vi "Lab Panel V5.0.vi"() -> ()   [LabVIEW 2013] (continued)
                      tunnel: w2669 -> [_ w2673]
                      frame False {
                      }
                      frame True {
                        n1581 = stacked-sequence {
                          tunnel: w2674 -> [w2677 _ _]
                          tunnel: w2673 -> [_ w2679 _]
                          frame #0 {
                            w2675 = FALSE
                            n1582 = local write "mail control"("END") -> ()
                            n1583 = Bundle(cluster=w2677) -> (w2678:T4)  [unwired: 3 in]
                            n1584 = local write "O/I  LAB05-1"(w2675) -> ()
                            n1585 = local write "RUN LAB05-1"(w2675) -> ()
                            n1586 = local write "run lab05-1"(w2675) -> ()
                            n1587 = local write "DISP LAB05-1"(w2678) -> ()
                          }
                          frame #1 {
                            n1588 = TDMS Close(11:w2679) -> (0:w2680:errorcluster)  [unwired: 1 in, 1 out]
                            n1589 = local write "data file error"(w2680) -> ()
                          }
                          frame #2 {
                            n1590 = stacked-sequence {
                              tunnel: "LAB05-1" -> [w2683 w2685]
                              frame #0 {
                                n1591 = call "sub vi - defrag tdms v1.vi"("panel id"=w2683) -> ("error out"=w2682:errorcluster)  [unwired: 10 in]
                                n1592 = local write "data file error"(w2682) -> ()
                              }
                              frame #1 {
                                n1593 = call "Save data file to network drive v2.vi"("panel id"=w2685) -> ("network file save error"=w2684:errorcluster)  [unwired: 9 in, 1 out]
                                n1594 = local write "data file error"(w2684) -> ()
                              }
                            }
                          }
                        }
                      }
                    }
                  }
                }
              }
              frame #9 {
                # "LAB05-2"
                n1595 = local read "run lab05-2"() -> (w2686:bool)
                n1596 = case shown="True" w2686 {
                  frame False {
                  }
                  frame True {
                    n1597 = local read "DISP LAB05-2"() -> (w2693:T4)
                    n1598 = Unbundle(w2693) -> ("CYCLE"=w2689:dbl, "STATUS"=w2694:string)  [unwired: 1 out]
                    n1599 = Not Equal?(x=w2694, y="RUN") -> (x != y?=w2688:bool)
                    n1600 = local read "TDMS LAB05-2"() -> (w2692:refnum<k34>)
                    n1601 = Greater?(x=w2689, y=2.0) -> (0:w2690:bool)
                    n1602 = And(x=w2690, y=w2688) -> (x .and. y?=w2687:bool)
                    n1603 = case shown="True" w2687 {
                      tunnel: w2693 -> [_ w2697]
                      tunnel: w2692 -> [_ w2696]
                      frame False {
                      }
                      frame True {
                        n1604 = stacked-sequence {
                          tunnel: w2697 -> [w2700 _ _]
                          tunnel: w2696 -> [_ w2702 _]
                          frame #0 {
                            w2698 = FALSE
                            n1605 = local write "mail control"("END") -> ()
                            n1606 = Bundle(cluster=w2700) -> (w2701:T4)  [unwired: 3 in]
                            n1607 = local write "RUN LAB05-2"(w2698) -> ()
                            n1608 = local write "O/I  LAB05-2"(w2698) -> ()
                            n1609 = local write "run lab05-2"(w2698) -> ()
                            n1610 = local write "DISP LAB05-2"(w2701) -> ()
                          }
                          frame #1 {
                            n1611 = TDMS Close(11:w2702) -> (0:w2703:errorcluster)  [unwired: 1 in, 1 out]
                            n1612 = local write "data file error"(w2703) -> ()
                          }
                          frame #2 {
                            n1613 = stacked-sequence {
                              tunnel: "LAB05-2" -> [w2706 w2708]
                              frame #0 {
                                n1614 = call "sub vi - defrag tdms v1.vi"("panel id"=w2706) -> ("error out"=w2705:errorcluster)  [unwired: 10 in]
                                n1615 = local write "data file error"(w2705) -> ()
                              }
                              frame #1 {
                                n1616 = call "Save data file to network drive v2.vi"("panel id"=w2708) -> ("network file save error"=w2707:errorcluster)  [unwired: 9 in, 1 out]
                                n1617 = local write "data file error"(w2707) -> ()
                              }
                            }
                          }
                        }
                      }
                    }
                  }
                }
              }
            }
            n1618 = local read "Network Directory"() -> (w2462:path)
            n1619 = global write "Global 1.vi" "Network Drive"(w2462) -> ()
          }
          frame #7 {
            # "disable functions"
            n1620 = stacked-sequence {
              tunnel: w2718 -> [w2732 _ w2789]
              tunnel: w2717 -> [w2727 _ w2788]
              tunnel: w2716 -> [w2726 _ w2787]
              tunnel: w2715 -> [w2724 _ w2786]
              tunnel: w2714 -> [w2725 _ w2785]
              tunnel: w2713 -> [_ w2749 w2784]
              tunnel: w2712 -> [_ w2750 w2783]
              tunnel: w2711 -> [_ w2751 w2782]
              tunnel: w2710 -> [_ w2752 w2781]
              tunnel: w2709 -> [_ w2753 w2780]
              frame #0 {
                n1621 = Select(t=2, s=w2724, f=0) -> (s? t:f=w2720:i32)
                n1622 = Select(t=2, s=w2726, f=0) -> (s? t:f=w2721:i32)
                n1623 = Select(t=2, s=w2725, f=0) -> (s? t:f=w2719:i32)
                n1624 = Select(t=2, s=w2732, f=0) -> (s? t:f=w2723:i32)
                n1625 = Select(t=2, s=w2727, f=0) -> (s? t:f=w2722:i32)
                n1626 = property on="SELECT LAB02-2" class="RadioBtnsControl (strict)"("DisabledEnum"=w2720) -> ()  [unwired: 2 in, 2 out]
                n1627 = property on="SELECT LAB02-1" class="RadioBtnsControl (strict)"("DisabledEnum"=w2721) -> ()  [unwired: 2 in, 2 out]
                n1628 = property on="SELECT LAB03-1" class="RadioBtnsControl (strict)"("DisabledEnum"=w2719) -> ()  [unwired: 2 in, 2 out]
                n1629 = property on="SELECT LAB01-1" class="RadioBtnsControl (strict)"("DisabledEnum"=w2723) -> ()  [unwired: 2 in, 2 out]
                n1630 = property on="SELECT LAB01-2" class="RadioBtnsControl (strict)"("DisabledEnum"=w2722) -> ()  [unwired: 2 in, 2 out]
                n1631 = Not(x=w2732) -> (.not. x?=w2733:bool)
                n1632 = property on="RESULT LAB01-1" class="Bool (strict)"("Visible"=w2733) -> ()  [unwired: 2 in, 2 out]
                n1633 = Not(x=w2727) -> (.not. x?=w2731:bool)
                n1634 = Not(x=w2726) -> (.not. x?=w2730:bool)
                n1635 = Not(x=w2724) -> (.not. x?=w2729:bool)
                n1636 = property on="RESULT LAB01-2" class="Bool (strict)"("Visible"=w2731) -> ()  [unwired: 2 in, 2 out]
                n1637 = Not(x=w2725) -> (.not. x?=w2728:bool)
                n1638 = property on="RESULT LAB02-1" class="Bool (strict)"("Visible"=w2730) -> ()  [unwired: 2 in, 2 out]
                n1639 = property on="RESULT LAB02-2" class="Bool (strict)"("Visible"=w2729) -> ()  [unwired: 2 in, 2 out]
                n1640 = property on="RESULT LAB03-1" class="Bool (strict)"("Visible"=w2728) -> ()  [unwired: 2 in, 2 out]
                n1641 = property on="SET LAB01-1" class="Clust (strict)"("DisabledEnum"=w2723) -> ()  [unwired: 2 in, 2 out]
                n1642 = property on="SET LAB01-2" class="Clust (strict)"("DisabledEnum"=w2722) -> ()  [unwired: 2 in, 2 out]
                n1643 = property on="SET LAB02-1" class="Clust (strict)"("DisabledEnum"=w2721) -> ()  [unwired: 2 in, 2 out]
                n1644 = property on="SET LAB02-2" class="Clust (strict)"("DisabledEnum"=w2720) -> ()  [unwired: 2 in, 2 out]
                n1645 = property on="SET LAB03-1" class="Clust (strict)"("DisabledEnum"=w2719) -> ()  [unwired: 2 in, 2 out]
                n1646 = property on="O/I  LAB01-1" class="Bool (strict)"("DisabledEnum"=w2723) -> ()  [unwired: 2 in, 2 out]
                n1647 = property on="O/I  LAB01-2" class="Bool (strict)"("DisabledEnum"=w2722) -> ()  [unwired: 2 in, 2 out]
                n1648 = property on="O/I  LAB02-1" class="Bool (strict)"("DisabledEnum"=w2721) -> ()  [unwired: 2 in, 2 out]
                n1649 = property on="O/I  LAB02-2" class="Bool (strict)"("DisabledEnum"=w2720) -> ()  [unwired: 2 in, 2 out]
                n1650 = property on="O/I  LAB03-1" class="Bool (strict)"("DisabledEnum"=w2719) -> ()  [unwired: 2 in, 2 out]
              }
              frame #1 {
                n1651 = Select(t=2, s=w2753, f=0) -> (s? t:f=w2744:i32)
                n1652 = Select(t=2, s=w2752, f=0) -> (s? t:f=w2745:i32)
                n1653 = Select(t=2, s=w2749, f=0) -> (s? t:f=w2748:i32)
                n1654 = Select(t=2, s=w2750, f=0) -> (s? t:f=w2747:i32)
                n1655 = Select(t=2, s=w2751, f=0) -> (s? t:f=w2746:i32)
                n1656 = property on="SELECT LAB05-2" class="RadioBtnsControl (strict)"("DisabledEnum"=w2744) -> ()  [unwired: 2 in, 2 out]
                n1657 = property on="SELECT LAB05-1" class="RadioBtnsControl (strict)"("DisabledEnum"=w2745) -> ()  [unwired: 2 in, 2 out]
                n1658 = property on="SELECT LAB03-2" class="RadioBtnsControl (strict)"("DisabledEnum"=w2748) -> ()  [unwired: 2 in, 2 out]
                n1659 = property on="SELECT LAB04-1" class="RadioBtnsControl (strict)"("DisabledEnum"=w2747) -> ()  [unwired: 2 in, 2 out]
                n1660 = property on="SELECT LAB04-2" class="RadioBtnsControl (strict)"("DisabledEnum"=w2746) -> ()  [unwired: 2 in, 2 out]
                n1661 = property on="SET LAB05-2" class="Clust (strict)"("DisabledEnum"=w2744) -> ()  [unwired: 2 in, 2 out]
                n1662 = property on="SET LAB05-1" class="Clust (strict)"("DisabledEnum"=w2745) -> ()  [unwired: 2 in, 2 out]
                n1663 = property on="SET LAB03-2" class="Clust (strict)"("DisabledEnum"=w2748) -> ()  [unwired: 2 in, 2 out]
                n1664 = property on="SET LAB04-1" class="Clust (strict)"("DisabledEnum"=w2747) -> ()  [unwired: 2 in, 2 out]
                n1665 = property on="SET LAB04-2" class="Clust (strict)"("DisabledEnum"=w2746) -> ()  [unwired: 2 in, 2 out]
                n1666 = property on="O/I  LAB05-2" class="Bool (strict)"("DisabledEnum"=w2744) -> ()  [unwired: 2 in, 2 out]
                n1667 = property on="O/I  LAB05-1" class="Bool (strict)"("DisabledEnum"=w2745) -> ()  [unwired: 2 in, 2 out]
                n1668 = property on="O/I  LAB04-1" class="Bool (strict)"("DisabledEnum"=w2747) -> ()  [unwired: 2 in, 2 out]
                n1669 = property on="O/I  LAB04-2" class="Bool (strict)"("DisabledEnum"=w2746) -> ()  [unwired: 2 in, 2 out]
                n1670 = property on="O/I  LAB03-2" class="Bool (strict)"("DisabledEnum"=w2748) -> ()  [unwired: 2 in, 2 out]
                n1671 = Not(x=w2753) -> (.not. x?=w2754:bool)
                n1672 = Not(x=w2752) -> (.not. x?=w2755:bool)
                n1673 = Not(x=w2751) -> (.not. x?=w2756:bool)
                n1674 = property on="RESULT LAB05-2" class="Bool (strict)"("Visible"=w2754) -> ()  [unwired: 2 in, 2 out]
                n1675 = property on="RESULT LAB05-1" class="Bool (strict)"("Visible"=w2755) -> ()  [unwired: 2 in, 2 out]
                n1676 = Not(x=w2750) -> (.not. x?=w2757:bool)
                n1677 = property on="RESULT LAB04-2" class="Bool (strict)"("Visible"=w2756) -> ()  [unwired: 2 in, 2 out]
                n1678 = Not(x=w2749) -> (.not. x?=w2758:bool)
                n1679 = property on="RESULT LAB04-1" class="Bool (strict)"("Visible"=w2757) -> ()  [unwired: 2 in, 2 out]
                n1680 = property on="RESULT LAB03-2" class="Bool (strict)"("Visible"=w2758) -> ()  [unwired: 2 in, 2 out]
              }
              frame #2 {
                # "disable calibrate if any test running"
                n1681 = Or(x=w2781, y=w2780) -> (x .or. y?=w2774:bool)
                n1682 = Or(x=w2783, y=w2782) -> (x .or. y?=w2776:bool)
                n1683 = Or(x=w2787, y=w2786) -> (x .or. y?=w2778:bool)
                n1684 = Or(x=w2785, y=w2784) -> (x .or. y?=w2777:bool)
                n1685 = Or(x=w2789, y=w2788) -> (x .or. y?=w2779:bool)
                n1686 = Or(x=w2777, y=w2776) -> (x .or. y?=w2775:bool)
                n1687 = Or(x=w2779, y=w2778) -> (x .or. y?=w2773:bool)
                n1688 = Or(x=w2775, y=w2774) -> (x .or. y?=w2772:bool)
                n1689 = Or(x=w2773, y=w2772) -> (x .or. y?=w2771:bool)
                n1690 = case shown="False" w2771 {
                  tunnel: [0 2] -> w2770
                  frame False {
                  }
                  frame True {
                  }
                }
                n1691 = property on="JIG TEST" class="Clust (strict)"("DisabledEnum"=w2770) -> ()  [unwired: 2 in, 2 out]
                n1692 = property on="Network Directory" class="Path"("DisabledEnum"=w2770) -> ()  [unwired: 2 in, 2 out]
                n1693 = property on="MAIL SETTINGS" class="Clust (strict)"("DisabledEnum"=w2770) -> ()  [unwired: 2 in, 2 out]
                n1694 = property on="SET (cal)" class="Bool (strict)"("DisabledEnum"=w2770) -> ()  [unwired: 2 in, 2 out]
                n1695 = property on="ADMIN" class="Bool (strict)"("DisabledEnum"=0) -> ()  [unwired: 2 in, 2 out]
              }
            }
          }
          frame #8 {
            # "drive jigs"
            n1696 = stacked-sequence {
              frame #0 {
                # "jig on"
                n1697 = local read "jig cycle"() -> (w2797:dbl)
                n1698 = property on="JIG TEST" class="Clust (strict)"() -> ("DisabledEnum"=w2794:T14)  [unwired: 2 in, 2 out]
                n1699 = Equal?(x=w2794, y=2) -> (x = y?=w2793:bool)
                n1700 = Equal?(x=w2797, y=0) -> (x = y?=w2795:bool)
                n1701 = And(x=w2795, y=w2793) -> (x .and. y?=w2792:bool)
                n1702 = case shown="True" w2792 {
                  frame False {
                  }
                  frame True {
                    n1703 = local read "run lab01-1"() -> (w2808:bool)
                    n1704 = local read "run lab01-2"() -> (w2807:bool)
                    n1705 = local read "run lab02-1"() -> (w2806:bool)
                    n1706 = local read "run lab02-2"() -> (w2805:bool)
                    n1707 = local read "run lab03-1"() -> (w2804:bool)
                    n1708 = local read "run lab03-2"() -> (w2803:bool)
                    n1709 = local read "run lab04-1"() -> (w2802:bool)
                    n1710 = local read "run lab04-2"() -> (w2801:bool)
                    n1711 = local read "run lab05-1"() -> (w2800:bool)
                    n1712 = local read "run lab05-2"() -> (w2799:bool)
                    n1713 = local write "JIG LAB03-2"(w2803) -> ()
                    n1714 = local write "JIG LAB01-1"(w2808) -> ()
                    n1715 = local write "JIG LAB01-2"(w2807) -> ()
                    n1716 = local write "JIG LAB02-1"(w2806) -> ()
                    n1717 = local write "JIG LAB02-2"(w2805) -> ()
                    n1718 = local write "JIG LAB03-1"(w2804) -> ()
                    n1719 = local write "JIG LAB04-1"(w2802) -> ()
                    n1720 = local write "JIG LAB04-2"(w2801) -> ()
                    n1721 = local write "JIG LAB05-1"(w2800) -> ()
                    n1722 = local write "JIG LAB05-2"(w2799) -> ()
                  }
                }
              }
              frame #1 {
                # "jig off"
                n1723 = local read "jig cycle"() -> (w2815:dbl)
                n1724 = local read "on loops"() -> (w2814:dbl)
                n1725 = property on="JIG TEST" class="Clust (strict)"() -> ("DisabledEnum"=w2813:T14)  [unwired: 2 in, 2 out]
                n1726 = Equal?(x=w2813, y=2) -> (x = y?=w2811:bool)
                n1727 = Equal?(x=w2815, y=w2814) -> (x = y?=w2810:bool)
                n1728 = And(x=w2810, y=w2811) -> (x .and. y?=w2809:bool)
                n1729 = case shown="True" w2809 {
                  frame False {
                  }
                  frame True {
                    w2866 = FALSE
                    w2867 = TRUE
                    w2865 = 2
                    n1730 = local read "SELECT LAB05-2"() -> (w2856:T3)
                    n1731 = local read "SELECT LAB04-2"() -> (w2858:T3)
                    n1732 = local read "SELECT LAB04-1"() -> (w2859:T3)
                    n1733 = local read "SELECT LAB05-1"() -> (w2857:T3)
                    n1734 = local read "SELECT LAB03-2"() -> (w2860:T3)
                    n1735 = local read "SELECT LAB02-1"() -> (w2863:T3)
                    n1736 = local read "SELECT LAB03-1"() -> (w2861:T3)
                    n1737 = local read "SELECT LAB02-2"() -> (w2862:T3)
                    n1738 = local read "SELECT LAB01-2"() -> (w2864:T3)
                    n1739 = local read "run lab05-1"() -> (w2826:bool)
                    n1740 = local read "run lab05-2"() -> (w2825:bool)
                    n1741 = local read "SELECT LAB01-1"() -> (w2868:T3)
                    n1742 = local read "run lab04-2"() -> (w2827:bool)
                    n1743 = local read "run lab04-1"() -> (w2828:bool)
                    n1744 = local read "run lab01-1"() -> (w2844:bool)
                    n1745 = local read "run lab01-2"() -> (w2833:bool)
                    n1746 = local read "run lab03-2"() -> (w2829:bool)
                    n1747 = local read "run lab03-1"() -> (w2830:bool)
                    n1748 = local read "run lab02-1"() -> (w2832:bool)
                    n1749 = local read "run lab02-2"() -> (w2831:bool)
                    n1750 = Equal?(x=w2865, y=w2861) -> (x = y?=w2839:bool)
                    n1751 = Equal?(x=w2865, y=w2860) -> (x = y?=w2838:bool)
                    n1752 = Equal?(x=w2865, y=w2859) -> (x = y?=w2837:bool)
                    n1753 = Equal?(x=w2865, y=w2858) -> (x = y?=w2836:bool)
                    n1754 = Equal?(x=w2865, y=w2857) -> (x = y?=w2835:bool)
                    n1755 = Equal?(x=w2865, y=w2856) -> (x = y?=w2834:bool)
                    n1756 = Equal?(x=w2865, y=w2868) -> (x = y?=w2845:bool)
                    n1757 = Equal?(x=w2865, y=w2863) -> (x = y?=w2841:bool)
                    n1758 = Equal?(x=w2865, y=w2862) -> (x = y?=w2840:bool)
                    n1759 = Equal?(x=w2865, y=w2864) -> (x = y?=w2842:bool)
                    n1760 = And(x=w2836, y=w2827) -> (x .and. y?=w2818:bool)
                    n1761 = And(x=w2839, y=w2830) -> (x .and. y?=w2821:bool)
                    n1762 = And(x=w2837, y=w2828) -> (x .and. y?=w2819:bool)
                    n1763 = And(x=w2834, y=w2825) -> (x .and. y?=w2816:bool)
                    n1764 = And(x=w2840, y=w2831) -> (x .and. y?=w2822:bool)
                    n1765 = And(x=w2838, y=w2829) -> (x .and. y?=w2820:bool)
                    n1766 = And(x=w2835, y=w2826) -> (x .and. y?=w2817:bool)
                    n1767 = And(x=w2842, y=w2833) -> (x .and. y?=w2824:bool)
                    n1768 = And(x=w2845, y=w2844) -> (x .and. y?=w2843:bool)
                    n1769 = And(x=w2841, y=w2832) -> (x .and. y?=w2823:bool)
                    n1770 = Select(t=w2867, s=w2843, f=w2866) -> (s? t:f=w2846:bool)
                    n1771 = Select(t=w2867, s=w2824, f=w2866) -> (s? t:f=w2847:bool)
                    n1772 = Select(t=w2867, s=w2823, f=w2866) -> (s? t:f=w2848:bool)
                    n1773 = Select(t=w2867, s=w2822, f=w2866) -> (s? t:f=w2849:bool)
                    n1774 = Select(t=w2867, s=w2821, f=w2866) -> (s? t:f=w2850:bool)
                    n1775 = Select(t=w2867, s=w2820, f=w2866) -> (s? t:f=w2851:bool)
                    n1776 = Select(t=w2867, s=w2819, f=w2866) -> (s? t:f=w2852:bool)
                    n1777 = Select(t=w2867, s=w2818, f=w2866) -> (s? t:f=w2853:bool)
                    n1778 = Select(t=w2867, s=w2817, f=w2866) -> (s? t:f=w2854:bool)
                    n1779 = Select(t=w2867, s=w2816, f=w2866) -> (s? t:f=w2855:bool)
                    n1780 = local write "JIG LAB03-2"(w2851) -> ()
                    n1781 = local write "JIG LAB02-1"(w2848) -> ()
                    n1782 = local write "JIG LAB02-2"(w2849) -> ()
                    n1783 = local write "JIG LAB01-2"(w2847) -> ()
                    n1784 = local write "JIG LAB03-1"(w2850) -> ()
                    n1785 = local write "JIG LAB01-1"(w2846) -> ()
                    n1786 = local write "JIG LAB05-2"(w2855) -> ()
                    n1787 = local write "JIG LAB04-1"(w2852) -> ()
                    n1788 = local write "JIG LAB05-1"(w2854) -> ()
                    n1789 = local write "JIG LAB04-2"(w2853) -> ()
                  }
                }
              }
            }
          }
          frame #9 {
            # "enable  jig test output if no test busy"
            n1790 = property on="JIG TEST" class="Clust (strict)"() -> ("DisabledEnum"=w2871:T14)  [unwired: 2 in, 2 out]
            n1791 = Equal?(x=w2871, y=0) -> (x = y?=w2869:bool)
            n1792 = case shown="True" w2869 {
              frame False {
              }
              frame True {
                n1793 = local read "JIG TEST"() -> (w2882:T9)
                n1794 = Unbundle(w2882) -> ("LAB01-1"=w2881:bool, "LAB01-2"=w2880:bool, "LAB02-1"=w2879:bool, "LAB02-2"=w2878:bool, "LAB03-1"=w2877:bool, "LAB03-2"=w2876:bool, "LAB04-1"=w2875:bool, "LAB04-2"=w2874:bool, "LAB05-1"=w2873:bool, "LAB05-2"=w2872:bool)
                n1795 = local write "JIG LAB05-1"(w2873) -> ()
                n1796 = local write "JIG LAB05-2"(w2872) -> ()
                n1797 = local write "JIG LAB04-1"(w2875) -> ()
                n1798 = local write "JIG LAB04-2"(w2874) -> ()
                n1799 = local write "JIG LAB03-2"(w2876) -> ()
                n1800 = local write "JIG LAB01-1"(w2881) -> ()
                n1801 = local write "JIG LAB02-1"(w2879) -> ()
                n1802 = local write "JIG LAB03-1"(w2877) -> ()
                n1803 = local write "JIG LAB01-2"(w2880) -> ()
                n1804 = local write "JIG LAB02-2"(w2878) -> ()
              }
            }
          }
          frame #10 {
            # "drive digital output"
            n1805 = local read "O/I  LAB05-2"() -> (w2889:bool)
            n1806 = local read "O/I  LAB05-1"() -> (w2891:bool)
            n1807 = local read "JIG LAB05-2"() -> (w2888:bool)
            n1808 = local read "O/I  LAB04-2"() -> (w2893:bool)
            n1809 = local read "JIG LAB05-1"() -> (w2890:bool)
            n1810 = local read "JIG LAB04-2"() -> (w2892:bool)
            n1811 = local read "O/I  LAB03-1"() -> (w2898:bool)
            n1812 = local read "O/I  LAB04-1"() -> (w2894:bool)
            n1813 = local read "O/I  LAB02-1"() -> (w2902:bool)
            n1814 = local read "O/I  LAB02-2"() -> (w2900:bool)
            n1815 = local read "O/I  LAB03-2"() -> (w2896:bool)
            n1816 = local read "JIG LAB04-1"() -> (w2887:bool)
            n1817 = local read "JIG LAB03-2"() -> (w2895:bool)
            n1818 = local read "O/I  LAB01-2"() -> (w2904:bool)
            n1819 = local read "JIG LAB02-1"() -> (w2901:bool)
            n1820 = local read "JIG LAB02-2"() -> (w2899:bool)
            n1821 = local read "JIG LAB03-1"() -> (w2897:bool)
            n1822 = local read "O/I  LAB01-1"() -> (w2906:bool)
            n1823 = local read "JIG LAB01-2"() -> (w2903:bool)
            n1824 = local read "JIG LAB01-1"() -> (w2905:bool)
            n1825 = Build Array(w2893, w2892, w2891, w2890, w2889, w2888) -> (w2884:bool[])
            n1826 = Build Array(w2899, w2898, w2897, w2896, w2895, w2894, w2887) -> (w2885:bool[])
            n1827 = Build Array(w2906, w2905, w2904, w2903, w2902, w2901, w2900) -> (w2886:bool[])
            n1828 = local read "simulate"() -> (w2883:bool)
            n1829 = case shown="False" w2883 {
              tunnel: w2886 -> [w2909 _]
              tunnel: w2885 -> [w2908 _]
              tunnel: w2884 -> [w2907 _]
              frame False {
                n1830 = call "sub vi - Drive Relays All v6.vi"("Array #2"=w2907, "Array #1"=w2908, "Array #0"=w2909) -> ()  [unwired: 8 in, 1 out]
              }
              frame True {
              }
            }
          }
          frame #11 {
            # "get analog values"
            n1831 = local read "on loops"() -> (w2916:dbl)
            n1832 = local read "jig cycle"() -> (w2913:dbl)
            n1833 = Add(x=w2916, y=1) -> (x+y=w2914:dbl)
            n1834 = Equal?(x=w2913, y=1) -> (x = y?=w2911:bool)
            n1835 = Equal?(x=w2913, y=w2914) -> (x = y?=w2912:bool)
            n1836 = Or(x=w2911, y=w2912) -> (x .or. y?=w2910:bool)
            n1837 = case shown="True" w2910 {
              frame False {
              }
              frame True {
                n1838 = local read "simulate"() -> (w2920:bool)
                n1839 = case shown="False" w2920 {
                  tunnel: [w2936 errorcluster[] [] ("array ERROR")] -> w2928
                  tunnel: [w2935 0.3 ("Analog loop time")] -> w2927
                  tunnel: [w2934 dynamicdata[] [] ("array GRAPH")] -> w2926
                  tunnel: [w2933 w2938] -> w2925
                  tunnel: [w2932 w2938] -> w2924
                  tunnel: [w2931 w2938] -> w2923
                  tunnel: [w2930 w2938] -> w2922
                  tunnel: [w2929 w2938] -> w2921
                  frame False {
                    n1840 = call "sub vi - Read Analog All v8.vi"() -> ("Analog loop time"=w2935:dbl, "array GRAPH"=w2934:dynamicdata[], "LAB01"=w2933:T23, "LAB02"=w2932:T24, "LAB03"=w2931:T25, "LAB04"=w2930:T26, "array ERROR"=w2936:errorcluster[], "LAB05"=w2929:T27)  [unwired: 7 in, 1 out]
                  }
                  frame True {
                    w2938 = T27 {"LAB05-1 (A)"=10.0, "LAB05-1 (V)"=220.0, "LAB05-1 (PF)"=0.5, "LAB05-2 (A)"=15.0, "LAB05-2 (V)"=225.0, "LAB05-2 (PF)"=0.6} ("LAB05")
                  }
                }
                n1841 = local read "simulate"() -> (w2919:bool)
                n1842 = stacked-sequence {
                  tunnel: w2928 -> [w2945 _ _ _ _ _]
                  tunnel: w2927 -> [w2944 _ _ _ _ _]
                  tunnel: w2926 -> [w2943 _ _ _ _ _]
                  tunnel: w2925 -> [_ w2992 _ _ _ _]
                  tunnel: w2924 -> [_ _ w2999 _ _ _]
                  tunnel: w2923 -> [_ _ _ w3028 _ _]
                  tunnel: w2922 -> [_ _ _ _ w3055 _]
                  tunnel: w2921 -> [_ _ _ _ _ w3084]
                  tunnel: w2919 -> [_ w2970 w2998 w3026 w3054 w3082]
                  tunnel: T12 {"1  (A) cal"=1.0, "1 (V) cal"=1.0, "1 (PF) cal"=1.0, "1 (TL) cal"=1.0, "1 (TN) cal"=1.0, "2 (A) cal"=1.0, "2 (V) cal"=1.0, "2 (PF) cal"=1.0, "2 (TL) cal"=1.0, "2 (TN) cal"=1.0} ("CAL LAB01") -> [_ w2969 w2997 w3025 w3053 w3081]
                  frame #0 {
                    n1843 = local write "AI"(TRUE) -> ()
                    n1844 = global write "Global 1.vi" "RATE(Hz)"("RATE (Hz)") -> ()
                    n1845 = global write "Global 1.vi" "SAMPLES"("SAMPLES") -> ()
                    n1846 = Index Array(array=w2943, index=6) -> (element=→"LAB04-1 (GRAPH)":dynamicdata)
                    n1847 = Index Array(array=w2943, index=7) -> (element=→"LAB04-2 (GRAPH)":dynamicdata)
                    n1848 = Index Array(array=w2943, index=9) -> (element=→"LAB05-2 (GRAPH)":dynamicdata)
                    n1849 = Index Array(array=w2943, index=8) -> (element=→"LAB05-1 (GRAPH)":dynamicdata)
                    n1850 = Index Array(array=w2943, index=5) -> (element=→"LAB03-2 (GRAPH)":dynamicdata)
                    n1851 = Index Array(array=w2943, index=0) -> (element=→"LAB01-1 (GRAPH)":dynamicdata)
                    n1852 = Index Array(array=w2943, index=1) -> (element=→"LAB01-2 (GRAPH)":dynamicdata)
                    n1853 = Index Array(array=w2943, index=2) -> (element=→"LAB02-1 (GRAPH)":dynamicdata)
                    n1854 = Index Array(array=w2943, index=3) -> (element=→"LAB02-2 (GRAPH)":dynamicdata)
                    n1855 = Index Array(array=w2943, index=4) -> (element=→"LAB03-1 (GRAPH)":dynamicdata)
                    "AI loop time" <- w2944
                    "Analog Error Array" <- w2945
                  }
                  frame #1 {
                    n1856 = Unbundle By Name(w2992) -> ("LAB05-1 (A)"=w2990:dbl, "LAB05-1 (V)"=w2989:dbl, "LAB05-1 (PF)"=w2988:dbl, "LAB05-2 (A)"=w2987:dbl, "LAB05-2 (V)"=w2986:dbl, "LAB05-2 (PF)"=w2985:dbl)
                    n1857 = case shown="False" w2970 {
                      tunnel: [w2993 w2994] -> w2991
                      tunnel: w2969 -> [_ w2994]
                      frame False {
                        n1858 = local read "CAL LAB01"() -> (w2993:T12)
                      }
                      frame True {
                      }
                    }
                    n1859 = Unbundle By Name(w2991) -> ("1  (A) cal"=w2984:dbl, "1 (V) cal"=w2983:dbl, "1 (PF) cal"=w2982:dbl, "2 (A) cal"=w2981:dbl, "2 (V) cal"=w2980:dbl, "2 (PF) cal"=w2979:dbl)  [unwired: 4 out]
                    n1860 = Multiply(x=w2990, y=w2984) -> (x*y=w2977:dbl)
                    n1861 = Multiply(x=w2989, y=w2983) -> (x*y=w2976:dbl)
                    n1862 = Multiply(x=w2988, y=w2982) -> (x*y=w2975:dbl)
                    n1863 = Multiply(x=w2987, y=w2981) -> (x*y=w2973:dbl)
                    n1864 = Multiply(x=w2986, y=w2980) -> (x*y=w2972:dbl)
                    n1865 = Multiply(x=w2985, y=w2979) -> (x*y=w2971:dbl)
                    n1866 = local read "SIG LAB01-1"() -> (w2978:T2)
                    n1867 = local read "SIG LAB01-2"() -> (w2974:T2)
                    n1868 = Bundle By Name(cluster=w2978, "AMPS"=w2977, "VOLTS"=w2976, "PF"=w2975) -> (w2968:T2)
                    n1869 = Bundle By Name(cluster=w2974, "AMPS"=w2973, "VOLTS"=w2972, "PF"=w2971) -> (w2967:T2)
                    n1870 = global write "Global display 1.vi" "SIG LAB01-2"(w2967) -> ()
                    n1871 = global write "Global display 1.vi" "SIG LAB01-1"(w2968) -> ()
                    n1872 = local write "SIG LAB01-2"(w2967) -> ()
                    n1873 = local write "SIG LAB01-1"(w2968) -> ()
                  }
                  frame #2 {
                    n1874 = Unbundle By Name(w2999) -> ("LAB05-1 (A)"=w3019:dbl, "LAB05-1 (V)"=w3018:dbl, "LAB05-1 (PF)"=w3017:dbl, "LAB05-2 (A)"=w3016:dbl, "LAB05-2 (V)"=w3015:dbl, "LAB05-2 (PF)"=w3014:dbl)
                    n1875 = case shown="True" w2998 {
                      tunnel: [w3021 w3022] -> w3020
                      tunnel: w2997 -> [_ w3022]
                      frame False {
                        n1876 = local read "CAL LAB02"() -> (w3021:T13)
                      }
                      frame True {
                      }
                    }
                    n1877 = Unbundle By Name(w3020) -> ("1  (A) cal"=w3013:dbl, "1 (V) cal"=w3012:dbl, "1 (PF) cal"=w3011:dbl, "2 (A) cal"=w3010:dbl, "2 (V) cal"=w3009:dbl, "2 (PF) cal"=w3008:dbl)  [unwired: 4 out]
                    n1878 = Multiply(x=w3019, y=w3013) -> (x*y=w3006:dbl)
                    n1879 = Multiply(x=w3018, y=w3012) -> (x*y=w3005:dbl)
                    n1880 = Multiply(x=w3017, y=w3011) -> (x*y=w3004:dbl)
                    n1881 = Multiply(x=w3016, y=w3010) -> (x*y=w3002:dbl)
                    n1882 = Multiply(x=w3015, y=w3009) -> (x*y=w3001:dbl)
                    n1883 = Multiply(x=w3014, y=w3008) -> (x*y=w3000:dbl)
                    n1884 = local read "SIG LAB02-1"() -> (w3007:T2)
                    n1885 = local read "SIG LAB02-2"() -> (w3003:T2)
                    n1886 = Bundle By Name(cluster=w3007, "AMPS"=w3006, "VOLTS"=w3005, "PF"=w3004) -> (w2996:T2)
                    n1887 = Bundle By Name(cluster=w3003, "AMPS"=w3002, "VOLTS"=w3001, "PF"=w3000) -> (w2995:T2)
                    n1888 = global write "Global display 1.vi" "SIG LAB02-1"(w2996) -> ()
                    n1889 = local write "SIG LAB02-2"(w2995) -> ()
                    n1890 = global write "Global display 1.vi" "SIG LAB02-2"(w2995) -> ()
                    n1891 = local write "SIG LAB02-1"(w2996) -> ()
                  }
                  frame #3 {
                    n1892 = Unbundle By Name(w3028) -> ("LAB05-1 (A)"=w3047:dbl, "LAB05-1 (V)"=w3046:dbl, "LAB05-1 (PF)"=w3045:dbl, "LAB05-2 (A)"=w3044:dbl, "LAB05-2 (V)"=w3043:dbl, "LAB05-2 (PF)"=w3042:dbl)
                    n1893 = case shown="True" w3026 {
                      tunnel: [w3049 w3050] -> w3048
                      tunnel: w3025 -> [_ w3050]
                      frame False {
                        n1894 = local read "CAL LAB03"() -> (w3049:T12)
                      }
                      frame True {
                      }
                    }
                    n1895 = Unbundle By Name(w3048) -> ("1  (A) cal"=w3041:dbl, "1 (V) cal"=w3040:dbl, "1 (PF) cal"=w3039:dbl, "2 (A) cal"=w3038:dbl, "2 (V) cal"=w3037:dbl, "2 (PF) cal"=w3036:dbl)  [unwired: 4 out]
                    n1896 = Multiply(x=w3047, y=w3041) -> (x*y=w3034:dbl)
                    n1897 = Multiply(x=w3046, y=w3040) -> (x*y=w3027:dbl)
                    n1898 = Multiply(x=w3045, y=w3039) -> (x*y=w3033:dbl)
                    n1899 = Multiply(x=w3044, y=w3038) -> (x*y=w3031:dbl)
                    n1900 = Multiply(x=w3043, y=w3037) -> (x*y=w3030:dbl)
                    n1901 = Multiply(x=w3042, y=w3036) -> (x*y=w3029:dbl)
                    n1902 = local read "SIG LAB03-1"() -> (w3035:T2)
                    n1903 = local read "SIG LAB03-2"() -> (w3032:T2)
                    n1904 = Bundle By Name(cluster=w3035, "AMPS"=w3034, "VOLTS"=w3027, "PF"=w3033) -> (w3024:T2)
                    n1905 = Bundle By Name(cluster=w3032, "AMPS"=w3031, "VOLTS"=w3030, "PF"=w3029) -> (w3023:T2)
                    n1906 = global write "Global display 1.vi" "SIG LAB03-1"(w3024) -> ()
                    n1907 = global write "Global display 1.vi" "SIG LAB03-2"(w3023) -> ()
                    n1908 = local write "SIG LAB03-2"(w3023) -> ()
                    n1909 = local write "SIG LAB03-1"(w3024) -> ()
                  }
                  frame #4 {
                    n1910 = Unbundle By Name(w3055) -> ("LAB05-1 (A)"=w3075:dbl, "LAB05-1 (V)"=w3074:dbl, "LAB05-1 (PF)"=w3073:dbl, "LAB05-2 (A)"=w3072:dbl, "LAB05-2 (V)"=w3071:dbl, "LAB05-2 (PF)"=w3070:dbl)
                    n1911 = case shown="False" w3054 {
                      tunnel: [w3077 w3078] -> w3076
                      tunnel: w3053 -> [_ w3078]
                      frame False {
                        n1912 = local read "CAL LAB04"() -> (w3077:T12)
                      }
                      frame True {
                      }
                    }
                    n1913 = Unbundle By Name(w3076) -> ("1  (A) cal"=w3069:dbl, "1 (V) cal"=w3068:dbl, "1 (PF) cal"=w3067:dbl, "2 (A) cal"=w3066:dbl, "2 (V) cal"=w3065:dbl, "2 (PF) cal"=w3064:dbl)  [unwired: 4 out]
                    n1914 = Multiply(x=w3075, y=w3069) -> (x*y=w3062:dbl)
                    n1915 = Multiply(x=w3074, y=w3068) -> (x*y=w3061:dbl)
                    n1916 = Multiply(x=w3073, y=w3067) -> (x*y=w3060:dbl)
                    n1917 = Multiply(x=w3072, y=w3066) -> (x*y=w3058:dbl)
                    n1918 = Multiply(x=w3071, y=w3065) -> (x*y=w3057:dbl)
                    n1919 = Multiply(x=w3070, y=w3064) -> (x*y=w3056:dbl)
                    n1920 = local read "SIG LAB04-1"() -> (w3063:T2)
                    n1921 = local read "SIG LAB04-2"() -> (w3059:T2)
                    n1922 = Bundle By Name(cluster=w3063, "AMPS"=w3062, "VOLTS"=w3061, "PF"=w3060) -> (w3052:T2)
                    n1923 = Bundle By Name(cluster=w3059, "AMPS"=w3058, "VOLTS"=w3057, "PF"=w3056) -> (w3051:T2)
                    n1924 = global write "Global display 1.vi" "SIG LAB04-2"(w3051) -> ()
                    n1925 = global write "Global display 1.vi" "SIG LAB04-1"(w3052) -> ()
                    n1926 = local write "SIG LAB04-2"(w3051) -> ()
                    n1927 = local write "SIG LAB04-1"(w3052) -> ()
                  }
                  frame #5 {
                    n1928 = Unbundle By Name(w3084) -> ("LAB05-1 (A)"=w3103:dbl, "LAB05-1 (V)"=w3083:dbl, "LAB05-1 (PF)"=w3102:dbl, "LAB05-2 (A)"=w3101:dbl, "LAB05-2 (V)"=w3100:dbl, "LAB05-2 (PF)"=w3099:dbl)
                    n1929 = case shown="False" w3082 {
                      tunnel: [w3105 w3106] -> w3104
                      tunnel: w3081 -> [_ w3106]
                      frame False {
                        n1930 = local read "CAL LAB05"() -> (w3105:T12)
                      }
                      frame True {
                      }
                    }
                    n1931 = Unbundle By Name(w3104) -> ("1  (A) cal"=w3098:dbl, "1 (V) cal"=w3097:dbl, "1 (PF) cal"=w3096:dbl, "2 (A) cal"=w3095:dbl, "2 (V) cal"=w3094:dbl, "2 (PF) cal"=w3093:dbl)  [unwired: 4 out]
                    n1932 = Multiply(x=w3103, y=w3098) -> (x*y=w3091:dbl)
                    n1933 = Multiply(x=w3083, y=w3097) -> (x*y=w3090:dbl)
                    n1934 = Multiply(x=w3102, y=w3096) -> (x*y=w3089:dbl)
                    n1935 = Multiply(x=w3101, y=w3095) -> (x*y=w3087:dbl)
                    n1936 = Multiply(x=w3100, y=w3094) -> (x*y=w3086:dbl)
                    n1937 = Multiply(x=w3099, y=w3093) -> (x*y=w3085:dbl)
                    n1938 = local read "SIG LAB05-1"() -> (w3092:T2)
                    n1939 = local read "SIG LAB05-2"() -> (w3088:T2)
                    n1940 = Bundle By Name(cluster=w3092, "AMPS"=w3091, "VOLTS"=w3090, "PF"=w3089) -> (w3080:T2)
                    n1941 = Bundle By Name(cluster=w3088, "AMPS"=w3087, "VOLTS"=w3086, "PF"=w3085) -> (w3079:T2)
                    n1942 = global write "Global display 1.vi" "SIG LAB05-1"(w3080) -> ()
                    n1943 = global write "Global display 1.vi" "SIG LAB05-2"(w3079) -> ()
                    n1944 = local write "SIG LAB05-2"(w3079) -> ()
                    n1945 = local write "SIG LAB05-1"(w3080) -> ()
                  }
                }
              }
            }
          }
          frame #12 {
            # "save test data to file"
            n1946 = Get Date/Time In Seconds() -> (seconds since 1Jan1904=w3107:timestamp)
            "File Time Stamp" <- w3107
            n1947 = local read "on loops"() -> (w3126:dbl)
            n1948 = local read "jig cycle"() -> (w3123:dbl)
            n1949 = Format Date/Time String(time format string (%c)="%H:%M%:%S", seconds (now)=w3107) -> (date/time string=w3111:string)  [unwired: 1 in]
            n1950 = Add(x=w3126, y=2) -> (x+y=w3124:dbl)
            n1951 = Build Array(w3111) -> (w3110:string[])
            n1952 = Equal?(x=w3123, y=1) -> (x = y?=w3109:bool)
            n1953 = Equal?(x=w3123, y=w3124) -> (x = y?=w3108:bool)
            n1954 = stacked-sequence {
              tunnel: w3122 -> [w3132 _ _ _ _ _ _ _ _ _]
              tunnel: w3121 -> [_ w3208 _ _ _ _ _ _ _ _]
              tunnel: w3120 -> [_ _ w3288 _ _ _ _ _ _ _]
              tunnel: w3119 -> [_ _ _ w3368 _ _ _ _ _ _]
              tunnel: w3118 -> [_ _ _ _ w3448 _ _ _ _ _]
              tunnel: w3117 -> [_ _ _ _ _ w3528 _ _ _ _]
              tunnel: w3116 -> [_ _ _ _ _ _ w3608 _ _ _]
              tunnel: w3115 -> [_ _ _ _ _ _ _ w3688 _ _]
              tunnel: w3114 -> [_ _ _ _ _ _ _ _ w3768 _]
              tunnel: w3113 -> [_ _ _ _ _ _ _ _ _ w3848]
              tunnel: w3110 -> [w3131 w3212 w3292 w3372 w3452 w3532 w3612 w3692 w3772 w3852]
              tunnel: w3109 -> [w3130 w3211 w3291 w3371 w3451 w3531 w3611 w3691 w3771 w3851]
              tunnel: w3108 -> [w3129 w3210 w3290 w3370 w3450 w3530 w3610 w3690 w3770 w3850]
              tunnel: w3107 -> [w3128 w3209 w3289 w3369 w3449 w3529 w3609 w3689 w3769 w3849]
              frame #0 {
                n1955 = case shown="True" w3132 {
                  tunnel: w3131 -> [_ w3137]
                  tunnel: w3130 -> [_ w3136]
                  tunnel: w3129 -> [_ w3134]
                  tunnel: w3128 -> [_ w3133]
                  frame False {
                  }
                  frame True {
                    n1956 = local read "DISP LAB01-1"() -> (w3138:T4)
                    n1957 = local read "SIG LAB01-1"() -> (w3139:T2)
                    n1958 = local read "ON L01-1"() -> (w3135:cluster{"amps":dbl, "volts":dbl, "pf":dbl})
                    n1959 = Unbundle(w3139) -> ("AMPS"=w3145:dbl, "VOLTS"=w3143:dbl, "PF"=w3142:dbl, "Tmp Live"=w3141:dbl, "Tmp Neut"=w3144:dbl)
                    n1960 = Unbundle(w3138) -> ("CYCLE"=w3140:dbl)  [unwired: 2 out]
                    n1961 = stacked-sequence {
                      tunnel: w3145 -> [w3149 w3168]
                      tunnel: w3144 -> [_ w3167]
                      tunnel: w3143 -> [w3148 w3166]
                      tunnel: w3142 -> [w3147 w3165]
                      tunnel: w3141 -> [_ w3164]
                      tunnel: w3140 -> [_ w3163]
                      tunnel: w3137 -> [_ w3162]
                      tunnel: w3136 -> [w3150 _]
                      tunnel: w3135 -> [w3146 w3160]
                      tunnel: w3134 -> [_ w3161]
                      tunnel: w3133 -> [_ w3156]
                      frame #0 {
                        n1962 = case shown="True" w3150 {
                          tunnel: w3149 -> [_ w3155]
                          tunnel: w3148 -> [_ w3154]
                          tunnel: w3147 -> [_ w3153]
                          tunnel: w3146 -> [_ w3151]
                          frame False {
                          }
                          frame True {
                            n1963 = Bundle(cluster=w3151, "amps"=w3155, "volts"=w3154, "pf"=w3153) -> (w3152:cluster{"amps":dbl, "volts":dbl, "pf":dbl})
                            n1964 = local write "ON L01-1"(w3152) -> ()
                          }
                        }
                      }
                      frame #1 {
                        n1965 = Unbundle(w3160) -> ("amps"=w3159:dbl, "volts"=w3158:dbl, "pf"=w3157:dbl)
                        n1966 = case shown="True" w3161 {
                          tunnel: w3168 -> [_ w3169]
                          tunnel: w3167 -> [_ w3207]
                          tunnel: w3166 -> [_ _]
                          tunnel: w3165 -> [_ _]
                          tunnel: w3164 -> [_ w3206]
                          tunnel: w3163 -> [_ w3205]
                          tunnel: w3162 -> [_ w3173]
                          tunnel: w3159 -> [_ w3170]
                          tunnel: w3158 -> [_ w3202]
                          tunnel: w3157 -> [_ w3201]
                          tunnel: w3156 -> [_ w3171]
                          frame False {
                          }
                          frame True {
                            n1967 = local read "TDMS LAB01-1"() -> (w3204:refnum<k34>)
                            n1968 = Build Array(w3202) -> (w3198:dbl[])
                            n1969 = Build Array(w3201) -> (w3197:dbl[])
                            n1970 = Build Array(w3206) -> (w3196:dbl[])
                            n1971 = Build Array(w3207) -> (w3195:dbl[])
                            n1972 = Build Array(w3170) -> (w3200:dbl[])
                            n1973 = Build Array(w3169) -> (w3199:dbl[])
                            n1974 = Build Array(w3205) -> (w3194:dbl[])
                            n1975 = Build Array("AMPS ON", "AMPS OFF", "VOLTS", "PF", "TEMP Live", "TEMP Neut", "CYCLE") -> (w3178:string[])
                            n1976 = Bundle By Name("Y"=w3200, "t0"=w3171) -> (w3193:waveform(dbl))  [unwired: 1 in]
                            n1977 = Bundle By Name("Y"=w3199, "t0"=w3171) -> (w3192:waveform(dbl))  [unwired: 1 in]
                            n1978 = Bundle By Name("Y"=w3198, "t0"=w3171) -> (w3191:waveform(dbl))  [unwired: 1 in]
                            n1979 = Bundle By Name("Y"=w3197, "t0"=w3171) -> (w3190:waveform(dbl))  [unwired: 1 in]
                            n1980 = Bundle By Name("Y"=w3196, "t0"=w3171) -> (w3189:waveform(dbl))  [unwired: 1 in]
                            n1981 = Bundle By Name("Y"=w3195, "t0"=w3171) -> (w3188:waveform(dbl))  [unwired: 1 in]
                            n1982 = Bundle By Name("Y"=w3194, "t0"=w3171) -> (w3187:waveform(dbl))  [unwired: 1 in]
                            n1983 = Build Array(w3193, w3192, w3191, w3190, w3189, w3188, w3187) -> (w3186:waveform(dbl)[])
                            n1984 = TDMS Write(0:w3204, 5:"TEST VALUES", 7:w3178, 9:w3186) -> (4:w3177:refnum<k34>, 6:w3176:string, 15:w3175:errorcluster)  [unwired: 2 in, 1 out]
                            n1985 = TDMS Write(0:w3177, 5:w3176, 7:"TIME", 9:w3173, 11:w3175) -> (15:w3172:errorcluster)  [unwired: 1 in, 3 out]
                            n1986 = local write "data file error"(w3172) -> ()
                          }
                        }
                      }
                    }
                  }
                }
              }
              frame #1 {
                n1987 = case shown="True" w3208 {
                  tunnel: w3212 -> [_ w3217]
                  tunnel: w3211 -> [_ w3216]
                  tunnel: w3210 -> [_ w3214]
                  tunnel: w3209 -> [_ w3213]
                  frame False {
                  }
                  frame True {
                    n1988 = local read "DISP LAB01-2"() -> (w3218:T4)
                    n1989 = local read "SIG LAB01-2"() -> (w3219:T2)
                    n1990 = local read "ON L01-2"() -> (w3215:cluster{"amps":dbl, "volts":dbl, "pf":dbl})
                    n1991 = Unbundle(w3219) -> ("AMPS"=w3225:dbl, "VOLTS"=w3223:dbl, "PF"=w3222:dbl, "Tmp Live"=w3221:dbl, "Tmp Neut"=w3224:dbl)
                    n1992 = Unbundle(w3218) -> ("CYCLE"=w3220:dbl)  [unwired: 2 out]
                    n1993 = stacked-sequence {
                      tunnel: w3225 -> [w3229 w3248]
                      tunnel: w3224 -> [_ w3247]
                      tunnel: w3223 -> [w3228 w3246]
                      tunnel: w3222 -> [w3227 w3245]
                      tunnel: w3221 -> [_ w3244]
                      tunnel: w3220 -> [_ w3243]
                      tunnel: w3217 -> [_ w3242]
                      tunnel: w3216 -> [w3230 _]
                      tunnel: w3215 -> [w3226 w3240]
                      tunnel: w3214 -> [_ w3241]
                      tunnel: w3213 -> [_ w3236]
                      frame #0 {
                        n1994 = case shown="True" w3230 {
                          tunnel: w3229 -> [_ w3235]
                          tunnel: w3228 -> [_ w3234]
                          tunnel: w3227 -> [_ w3233]
                          tunnel: w3226 -> [_ w3231]
                          frame False {
                          }
                          frame True {
                            n1995 = Bundle(cluster=w3231, "amps"=w3235, "volts"=w3234, "pf"=w3233) -> (w3232:cluster{"amps":dbl, "volts":dbl, "pf":dbl})
                            n1996 = local write "ON L01-2"(w3232) -> ()
                          }
                        }
                      }
                      frame #1 {
                        n1997 = Unbundle(w3240) -> ("amps"=w3239:dbl, "volts"=w3238:dbl, "pf"=w3237:dbl)
                        n1998 = case shown="True" w3241 {
                          tunnel: w3248 -> [_ w3280]
                          tunnel: w3247 -> [_ w3287]
                          tunnel: w3246 -> [_ _]
                          tunnel: w3245 -> [_ _]
                          tunnel: w3244 -> [_ w3286]
                          tunnel: w3243 -> [_ w3285]
                          tunnel: w3242 -> [_ w3250]
                          tunnel: w3239 -> [_ w3282]
                          tunnel: w3238 -> [_ w3281]
                          tunnel: w3237 -> [_ w3279]
                          tunnel: w3236 -> [_ w3271]
                          frame False {
                          }
                          frame True {
                            n1999 = local read "TDMS LAB01-2"() -> (w3284:refnum<k34>)
                            n2000 = Build Array(w3281) -> (w3276:dbl[])
